vi "Get_Dust_Info_for_Live_Plot.vi"(3 "error in (no error)":errorcluster) -> (5 "Dust Event":T1 {"File Location" items=["Unknown"=-5, "IDL Processing"=-4, "Writing from Queue"=-3, "Labview Files"=-2, "Retry Labview files"=-1, "Local Cache "=0, "Storage"=1]}, 6 "Experiment Name":string, 7 "Dust Density":dbl, 8 "Dust Type":string, 9 "Group Name":string, 10 "error out":errorcluster)   [LabVIEW 2013]
uses:
  Public API/Post_Dust_Event.ctl
  File_location.ctl
  <vilib>/addons/database/Connection.llb/Conn Execute.vi
  <vilib>/addons/database/Recordset.llb/Rec Fetch Recordset Data (R).vi
  <vilib>/addons/database/Recordset.llb/Rec Destroy - Connection.vi
  <vilib>/addons/database/_DB Variant To Data/Database Variant To Data.xnode
  <vilib>/addons/database/NI_Database_API.lvlib
panel:
  # "Dust Event"
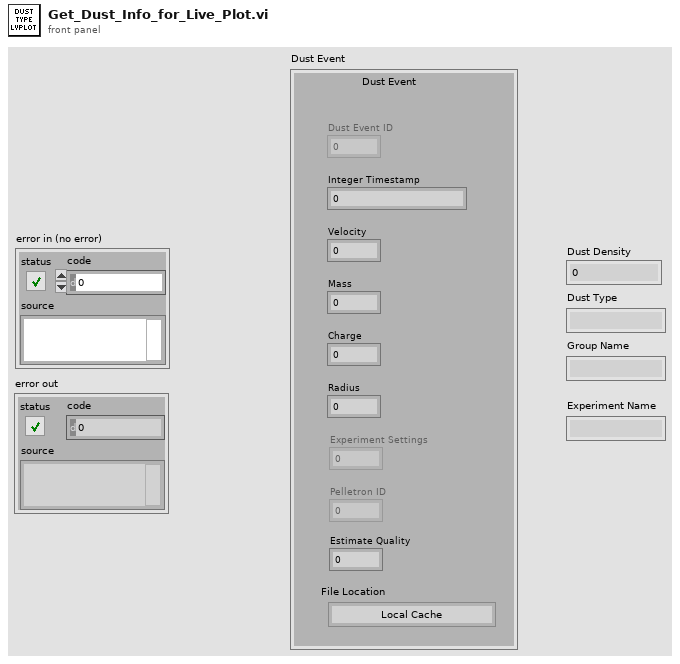
[diagram p1: front panel]
types:
  T1 = typedef "Post_Dust_Event.ctl" = cluster{"Dust Event ID":i64, "Integer Timestamp":i64, "Velocity":sgl, "Mass":sgl, "Charge":sgl, "Radius":sgl, "Experiment Settings":dbl, "Pelletron ID":i32, "Estimate Quality":sgl, "File Location":T2, "id_dust_info":dbl}
  T2 = typedef "File_location.ctl" = i8
  T3 = typedef "NI_Database_API.lvlib/Conn ObjectReference.ctl" = refnum<k1>
  T4 = typedef "NI_Database_API.lvlib/Rec ObjectReference.ctl" = refnum<k1>
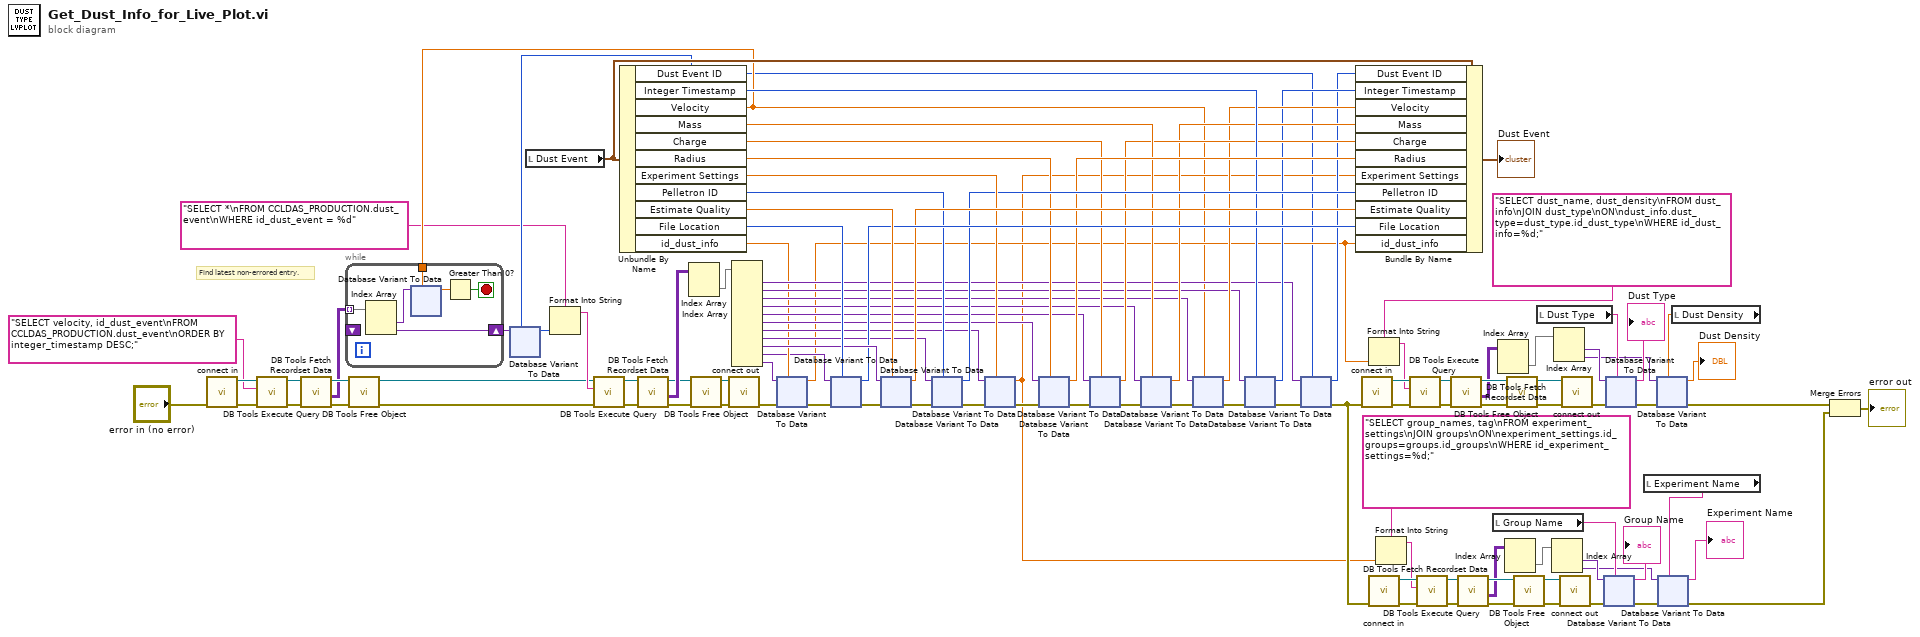
[diagram p0: block diagram]
diagram:
  # "Find latest non-errored entry."
  n1 = call "connect in.vi"("error in (no error)"="error in (no error)") -> ("error out"=w25:errorcluster, "Database Connection"=w24:T3)  [unwired: 6 in, 1 out]
  n2 = call-poly <vilib>:"DB Tools Execute Query.vi"("error in (no error)"=w25, "SQL query"="SELECT velocity, id_dust_event\nFROM CCLDAS_PRODUCTION.dust_event\nORDER BY integer_timestamp DESC;" ("format string"), "connection reference"=w24) -> ("error out"=w20:errorcluster, "recordset reference"=w23:T4)  [unwired: 5 in]
  n3 = call-poly <vilib>:"DB Tools Fetch Recordset Data.vi"("error in (no error)"=w20, "recordset reference"=w23) -> ("error out"=w21:errorcluster, "recordset data"=w18:variant[][], "recordset reference out"=w22:T4)  [unwired: 3 in]
  n4 = call-poly <vilib>:"DB Tools Free Object.vi"("error in (no error)"=w21, "recordset reference"=w22) -> ("error out"=w11:errorcluster, "connection reference"=w10:T3)  [unwired: 8 in]
  n5 = local read "Dust Event"() -> (w102:T1)
  n6 = Unbundle By Name(w102) -> ("Dust Event ID"=w15:i64, "Integer Timestamp"=w78:i64, "Velocity"=w17:sgl, "Mass"=w81:sgl, "Charge"=w82:sgl, "Radius"=w87:sgl, "Experiment Settings"=w92:dbl, "Pelletron ID"=w95:i32, "Estimate Quality"=w98:sgl, "File Location"=w103:T2, "id_dust_info"=w63:dbl)
  n7 = while {
    tunnel: w18 -> [w119] mode=indexing
    tunnel: w17 -> [w118]
    shift-right: [w116] -> w16
    shift-left: _ -> [_]
    stop <- w114 stop-if-true
    n8 = Index Array(array=w119) -> (element #1=w117:variant, element #2=w116:variant)  [unwired: 2 in]
    n9 = xnode "Database Variant To Data"("database variant"=w117, "type"=w118) -> ("data"=w115:sgl)  [unwired: 1 in, 1 out]
    n10 = Greater Than 0?(x=w115) -> (x > 0?=w114:bool)
  }
  n11 = xnode "Database Variant To Data"("database variant"=w16, "type"=w15) -> ("data"=w12:i64)  [unwired: 1 in, 1 out]
  n12 = Format Into String(format string="SELECT *\nFROM CCLDAS_PRODUCTION.dust_event\nWHERE id_dust_event = %d", w12) -> (resulting string=w13:string)  [unwired: 2 in, 1 out]
  n13 = call-poly <vilib>:"DB Tools Execute Query.vi"("error in (no error)"=w11, "SQL query"=w13, "connection reference"=w10) -> ("error out"=w29:errorcluster, "recordset reference"=w30:T4)  [unwired: 5 in]
  n14 = call-poly <vilib>:"DB Tools Fetch Recordset Data.vi"("error in (no error)"=w29, "recordset reference"=w30) -> ("error out"=w28:errorcluster, "recordset data"=w33:variant[][], "recordset reference out"=w32:T4)  [unwired: 3 in]
  n15 = Index Array(array=w33) -> (element=w113:variant[])  [unwired: 2 in]
  n16 = call-poly <vilib>:"DB Tools Free Object.vi"("error in (no error)"=w28, "recordset reference"=w32) -> ("error out"=w27:errorcluster, "connection reference"=w31:T3)  [unwired: 8 in]
  n17 = call "connect out.vi"("error in (no error)"=w27, "connection reference"=w31) -> ("error out"=w65:errorcluster)  [unwired: 9 in]
  n18 = Index Array(array=w113) -> (element #1=w68:variant, element #2=w69:variant, element #3=w70:variant, element #4=w71:variant, element #5=w84:variant, element #6=w88:variant, element #7=w90:variant, element #8=w94:variant, element #9=w100:variant, element #10=w62:variant, element #11=w64:variant)  [unwired: 11 in]
  n19 = xnode "Database Variant To Data"("database variant"=w64, "error in (no error)"=w65, "type"=w63) -> ("data"=w61:dbl, "error out"=w66:errorcluster)
  n20 = xnode "Database Variant To Data"("database variant"=w62, "error in (no error)"=w66, "type"=w103) -> ("data"=w97:T2, "error out"=w101:errorcluster)
  n21 = xnode "Database Variant To Data"("database variant"=w100, "error in (no error)"=w101, "type"=w98) -> ("data"=w96:sgl, "error out"=w99:errorcluster)
  n22 = xnode "Database Variant To Data"("database variant"=w94, "error in (no error)"=w99, "type"=w95) -> ("data"=w91:i32, "error out"=w93:errorcluster)
  n23 = xnode "Database Variant To Data"("database variant"=w90, "error in (no error)"=w93, "type"=w92) -> ("data"=w46:dbl, "error out"=w89:errorcluster)
  n24 = xnode "Database Variant To Data"("database variant"=w88, "error in (no error)"=w89, "type"=w87) -> ("data"=w85:sgl, "error out"=w86:errorcluster)
  n25 = xnode "Database Variant To Data"("database variant"=w84, "error in (no error)"=w86, "type"=w82) -> ("data"=w76:sgl, "error out"=w83:errorcluster)
  n26 = xnode "Database Variant To Data"("database variant"=w71, "error in (no error)"=w83, "type"=w81) -> ("data"=w75:sgl, "error out"=w80:errorcluster)
  n27 = xnode "Database Variant To Data"("database variant"=w70, "error in (no error)"=w80, "type"=w17) -> ("data"=w74:sgl, "error out"=w79:errorcluster)
  n28 = xnode "Database Variant To Data"("database variant"=w69, "error in (no error)"=w79, "type"=w78) -> ("data"=w73:i64, "error out"=w77:errorcluster)
  n29 = xnode "Database Variant To Data"("database variant"=w68, "error in (no error)"=w77, "type"=w15) -> ("data"=w72:i64, "error out"=w47:errorcluster)
  n30 = Bundle By Name(cluster=w102, "Dust Event ID"=w72, "Integer Timestamp"=w73, "Velocity"=w74, "Mass"=w75, "Charge"=w76, "Radius"=w85, "Experiment Settings"=w46, "Pelletron ID"=w91, "Estimate Quality"=w96, "File Location"=w97, "id_dust_info"=w61) -> (→"Dust Event":T1)
  n31 = call "connect in.vi"("error in (no error)"=w47) -> ("error out"=w112:errorcluster, "Database Connection"=w107:T3)  [unwired: 6 in, 1 out]
  n32 = Format Into String(format string="SELECT dust_name, dust_density\nFROM dust_info\nJOIN dust_type\nON\ndust_info.dust_type=dust_type.id_dust_type\nWHERE id_dust_info=%d;", w61) -> (resulting string=w106:string)  [unwired: 2 in, 1 out]
  n33 = call "connect in.vi"("error in (no error)"=w47) -> ("error out"=w56:errorcluster, "Database Connection"=w51:T3)  [unwired: 6 in, 1 out]
  n34 = Format Into String(format string="SELECT group_names, tag\nFROM experiment_settings\nJOIN groups\nON\nexperiment_settings.id_groups=groups.id_groups\nWHERE id_experiment_settings=%d;", w46) -> (resulting string=w50:string)  [unwired: 2 in, 1 out]
  n35 = call-poly <vilib>:"DB Tools Execute Query.vi"("error in (no error)"=w112, "SQL query"=w106, "connection reference"=w107) -> ("error out"=w111:errorcluster, "recordset reference"=w108:T4)  [unwired: 5 in]
  n36 = call-poly <vilib>:"DB Tools Execute Query.vi"("error in (no error)"=w56, "SQL query"=w50, "connection reference"=w51) -> ("error out"=w55:errorcluster, "recordset reference"=w52:T4)  [unwired: 5 in]
  n37 = call-poly <vilib>:"DB Tools Fetch Recordset Data.vi"("error in (no error)"=w111, "recordset reference"=w108) -> ("error out"=w109:errorcluster, "recordset data"=w104:variant[][], "recordset reference out"=w110:T4)  [unwired: 3 in]
  n38 = call-poly <vilib>:"DB Tools Fetch Recordset Data.vi"("error in (no error)"=w55, "recordset reference"=w52) -> ("error out"=w53:errorcluster, "recordset data"=w48:variant[][], "recordset reference out"=w54:T4)  [unwired: 3 in]
  n39 = local read "Group Name"() -> (w42:string)
  n40 = Index Array(array=w104) -> (element=w39:variant[])  [unwired: 2 in]
  n41 = Index Array(array=w48) -> (element=w36:variant[])  [unwired: 2 in]
  n42 = call-poly <vilib>:"DB Tools Free Object.vi"("error in (no error)"=w109, "recordset reference"=w110) -> ("error out"=w38:errorcluster, "connection reference"=w37:T3)  [unwired: 8 in]
  n43 = call-poly <vilib>:"DB Tools Free Object.vi"("error in (no error)"=w53, "recordset reference"=w54) -> ("error out"=w35:errorcluster, "connection reference"=w34:T3)  [unwired: 8 in]
  n44 = local read "Dust Type"() -> (w58:string)
  n45 = Index Array(array=w36) -> (element #1=w44:variant, element #2=w3:variant)  [unwired: 2 in]
  n46 = Index Array(array=w39) -> (element #1=w59:variant, element #2=w7:variant)  [unwired: 2 in]
  n47 = call "connect out.vi"("error in (no error)"=w35, "connection reference"=w34) -> ("error out"=w45:errorcluster)  [unwired: 9 in]
  n48 = call "connect out.vi"("error in (no error)"=w38, "connection reference"=w37) -> ("error out"=w60:errorcluster)  [unwired: 9 in]
  n49 = xnode "Database Variant To Data"("database variant"=w44, "error in (no error)"=w45, "type"=w42) -> ("data"=→"Group Name":string, "error out"=w40:errorcluster)
  n50 = xnode "Database Variant To Data"("database variant"=w59, "error in (no error)"=w60, "type"=w58) -> ("data"=→"Dust Type":string, "error out"=w9:errorcluster)
  n51 = local read "Experiment Name"() -> (w1:string)
  n52 = xnode "Database Variant To Data"("database variant"=w3, "error in (no error)"=w40, "type"=w1) -> ("data"=→"Experiment Name":string, "error out"=w4:errorcluster)
  n53 = local read "Dust Density"() -> (w5:dbl)
  n54 = xnode "Database Variant To Data"("database variant"=w7, "error in (no error)"=w9, "type"=w5) -> ("data"=→"Dust Density":dbl, "error out"=w8:errorcluster)
  n55 = Merge Errors(w8, w4) -> (→"error out":errorcluster)
